vi "CheckHeaderCode.vi"(8 "error in (no error)":errorcluster, 10 "Expected code (200)":T1=200 items=["200 OK"=200, "201 Created"=201, "400 Bad Request"=400, "401 Unauthorized"=401, "403 Forbidden"=403, "404 Not Found"=404, "405 Method Not Allowed"=405, "406 Not Acceptable"=406, "500 Internal Server Error"=500], 11 "Headers":string="HTTP/1.1 200 OK\r\nServer: nginx/1.17.6\r\nDate: Thu, 04 Nov 2021 12:06:49 GMT\r\nContent-Type: application/json\r\nContent-Length: 12191\r\nConnection: keep-alive\r\nVary: Accept-Encoding\r\nVary: Accept, Accept-Encoding, Accept-Language, Cookie\r\nAllow: GET, POST, HEAD, OPTIONS\r\nX-Frame-Options: DENY\r\nContent-Language: it\r\nX-Content-Type-Options: nosniff\r\nX-XSS-Protection: 1; mode=block\r\nCache-Control: no-cache=\"Set-Cookie\"\r\n\r\n") -> (0 "error out":errorcluster)   [LabVIEW 2019, in "ByteREST.lvlib" / "ByteRESTBase.lvclass"]
doc: "Cerca un determinato codice nella prima riga di Header, se non trova restituisce un errore \"BadResponse\""
uses:
  ByteRESTBase.lvclass
  Status_Code.ctl
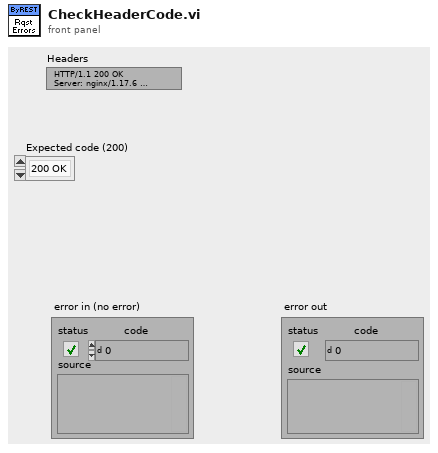
[diagram p1: front panel]
types:
  T1 = typedef "ByteREST.lvlib/ByteRESTBase.lvclass/Status_Code.ctl" = u16
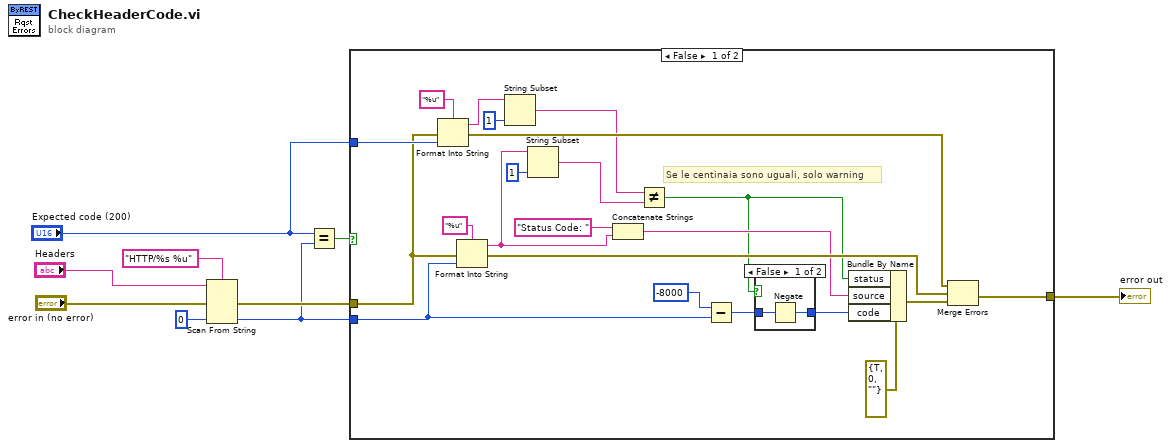
[diagram p0: block diagram]
diagram:
  n1 = Scan From String(format string="HTTP/%s %u", input string="Headers", error in="error in (no error)", default 2=u16 0) -> (error out=w4:errorcluster, output 2=w2:u16)  [unwired: 3 in, 2 out]
  n2 = Equal?(x="Expected code (200)", y=w2) -> (x = y?=w5:bool)
  n3 = case shown="False" w5 {
    tunnel: w4 -> [w18 w35]
    tunnel: [w27 w35] -> w3
    tunnel: w2 -> [w28 _]
    tunnel: "Expected code (200)" -> [w19 _]
    frame False {
      # "Se le centinaia sono uguali, solo warning"
      n4 = Format Into String(format string="%u", error in=w18, w19) -> (resulting string=w15:string, error out=w17:errorcluster)  [unwired: 1 in]
      n5 = Format Into String(format string="%u", error in=w18, w28) -> (resulting string=w22:string, error out=w25:errorcluster)  [unwired: 1 in]
      n6 = String Subset(string=w15, length (rest)=1 ("length (rest)")) -> (substring=w13:string)  [unwired: 1 in]
      n7 = String Subset(string=w22, length (rest)=1 ("length (rest)")) -> (substring=w14:string)  [unwired: 1 in]
      n8 = Concatenate Strings("Status Code: " ("initial string"), w22) -> (w23:string)
      n9 = Not Equal?(x=w13, y=w14) -> (x != y?=w10:bool)
      n10 = Subtract(x=-8000, y=w28) -> (x-y=w11:i32)
      n11 = case shown="False" w10 {
        tunnel: [w33 w34] -> w12
        tunnel: w11 -> [w32 w34]
        frame False {
          n12 = Negate(x=w32) -> (-x=w33:i32)
        }
        frame True {
        }
      }
      n13 = Bundle By Name(cluster=errorcluster {"status"=TRUE, "code"=0, "source"=""} ("error IO"), "status"=w10, "source"=w23, "code"=w12) -> (w26:errorcluster)
      n14 = Merge Errors(w17, w25, w26) -> (w27:errorcluster)
    }
    frame True {
    }
  }
  "error out" <- w3
